vi "ReadScaledAxis.vi"(8 "error in (no error)":errorcluster, 10 "Arduino Resource In":T1={"VISA resource"="", "Board Type"=enum."Uno", "Connection Type"=enum."USB / Serial", "Bytes Per Packet (15)"=15}, 11 "HMC5883L in":refnum<class "HMC5883L.lvclass">) -> (0 "error out":errorcluster, 2 "Arduino Resource out":T1={"VISA resource"="", "Board Type"=enum."Uno", "Connection Type"=enum."USB / Serial", "Bytes Per Packet (15)"=15}, 3 "HMC5883L out":refnum<class "HMC5883L.lvclass">)   [LabVIEW 2012, in "HMC5883L.lvclass"]
uses:
  HMC5883L.lvclass
  <vilib>/LabVIEW Interface for Arduino/Type Defs/Arduino Resource.ctl
  <vilib>/LabVIEW Interface for Arduino/Type Defs/Board Type.ctl
  HMC5883L.lvclass/HMC5883L.ctl
  <vilib>/LabVIEW Interface for Arduino/LabVIEW Interface for Arduino.lvlib
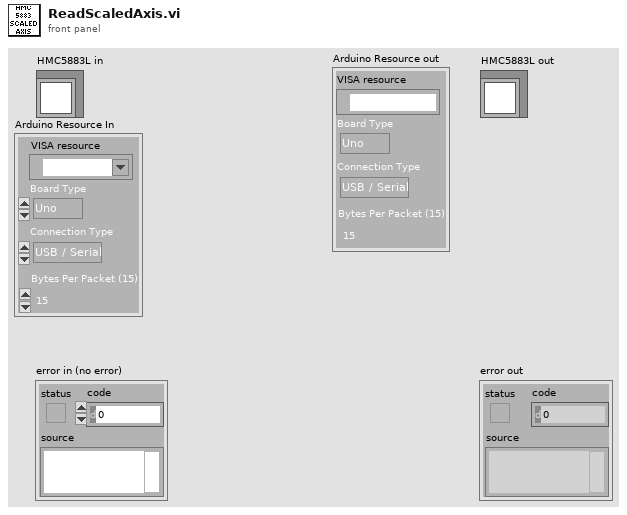
[diagram p1: front panel]
types:
  T1 = typedef "LabVIEW Interface for Arduino.lvlib/Arduino Resource.ctl" = cluster{"VISA resource":refnum<visa-resource-name>, "Board Type":T2, "Connection Type":enum8{"USB / Serial"}, "Bytes Per Packet (15)":u8}
  T2 = typedef "LabVIEW Interface for Arduino.lvlib/Board Type.ctl" = enum16{"Uno", "Dimuelanove w/Atmega 328", "Mega 2560"}
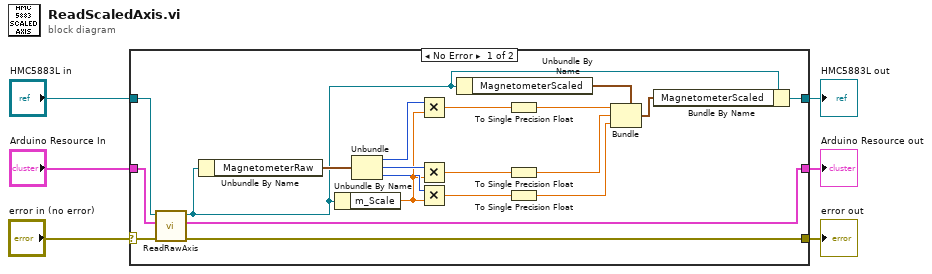
[diagram p0: block diagram]
diagram:
  n1 = case shown="No Error" "error in (no error)" {
    selector: "error in (no error)" -> [w8 w29]
    tunnel: [w7 w29] -> w5
    tunnel: [w12 w28] -> w3
    tunnel: "HMC5883L in" -> [w26 w28]
    tunnel: "Arduino Resource In" -> [w25 w27]
    tunnel: [w24 w27] -> w1
    frame No Error {
      n2 = call-dynamic "ReadRawAxis.vi"("error in (no error)"=w8, "Arduino Resource In"=w25, "HMC5883L in"=w26) -> ("error out"=w7:errorcluster, "Arduino Resource out"=w24:T1, "HMC5883L out"=w11:refnum<class "HMC5883L.lvclass">)  [unwired: 6 in]
      n3 = Unbundle By Name(w11) -> ("MagnetometerRaw"=w23:cluster{"XAxis":i16, "YAxis":i16, "ZAxis":i16})
      n4 = Unbundle By Name(w11) -> ("m_Scale"=w19:dbl)
      n5 = Unbundle(w23) -> ("XAxis"=w22:i16, "YAxis"=w21:i16, "ZAxis"=w20:i16)
      n6 = Multiply(x=w22, y=w19) -> (x*y=w18:dbl)
      n7 = Multiply(x=w21, y=w19) -> (x*y=w16:dbl)
      n8 = Multiply(x=w20, y=w19) -> (x*y=w17:dbl)
      n9 = Unbundle By Name(w11) -> ("MagnetometerScaled"=w10:cluster{"XAxis":sgl, "YAxis":sgl, "ZAxis":sgl})
      n10 = To Single Precision Float(number=w18) -> (single precision float=w15:sgl)
      n11 = To Single Precision Float(number=w16) -> (single precision float=w14:sgl)
      n12 = To Single Precision Float(number=w17) -> (single precision float=w13:sgl)
      n13 = Bundle(cluster=w10, "XAxis"=w15, "YAxis"=w14, "ZAxis"=w13) -> (w9:cluster{"XAxis":sgl, "YAxis":sgl, "ZAxis":sgl})
      n14 = Bundle By Name(cluster=w11, "MagnetometerScaled"=w9) -> (w12:refnum<class "HMC5883L.lvclass">)
    }
    frame Error {
    }
  }
  "error out" <- w5
  "HMC5883L out" <- w3
  "Arduino Resource out" <- w1
